vi "PIDRelay.vi"() -> ()   [LabVIEW 2020]
uses:
  <vilib>/Instr/_visa.llb/VISA Configure Serial Port (Instr).vi
  <vilib>/addons/control/pid/NI_PID_pid.lvlib
  <vilib>/addons/control/pid/pid.llb/PID (DBL).vi
panel:
  in  "setpoint":dbl format="%.2f"
  in  "process variable":dbl format="%.2f"
  in  "PID gains":T1={"proportional gain (Kc)"=1.0, "integral time (Ti, min)"=0.01, "derivative time (Td, min)"=0.0} {"derivative time (Td, min)" format="%.3f"; "integral time (Ti, min)" format="%.3f"; "proportional gain (Kc)" format="%.3f"}
  in  "dt (s)":dbl=-1.0 format="%.3f"
  in  "output range":cluster{"output high":dbl, "output low":dbl}={"output high"=100.0, "output low"=-100.0} {"output low" format="%.2f"; "output high" format="%.2f"}
  in  "VISA resource name 2":refnum<visa-resource-name>
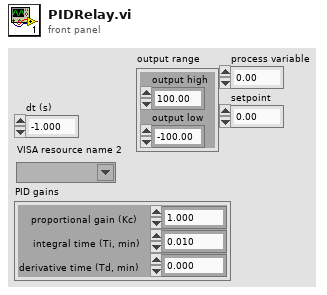
[diagram p1: front panel]
types:
  T1 = cluster{"proportional gain (Kc)":dbl, "integral time (Ti, min)":dbl, "derivative time (Td, min)":dbl}
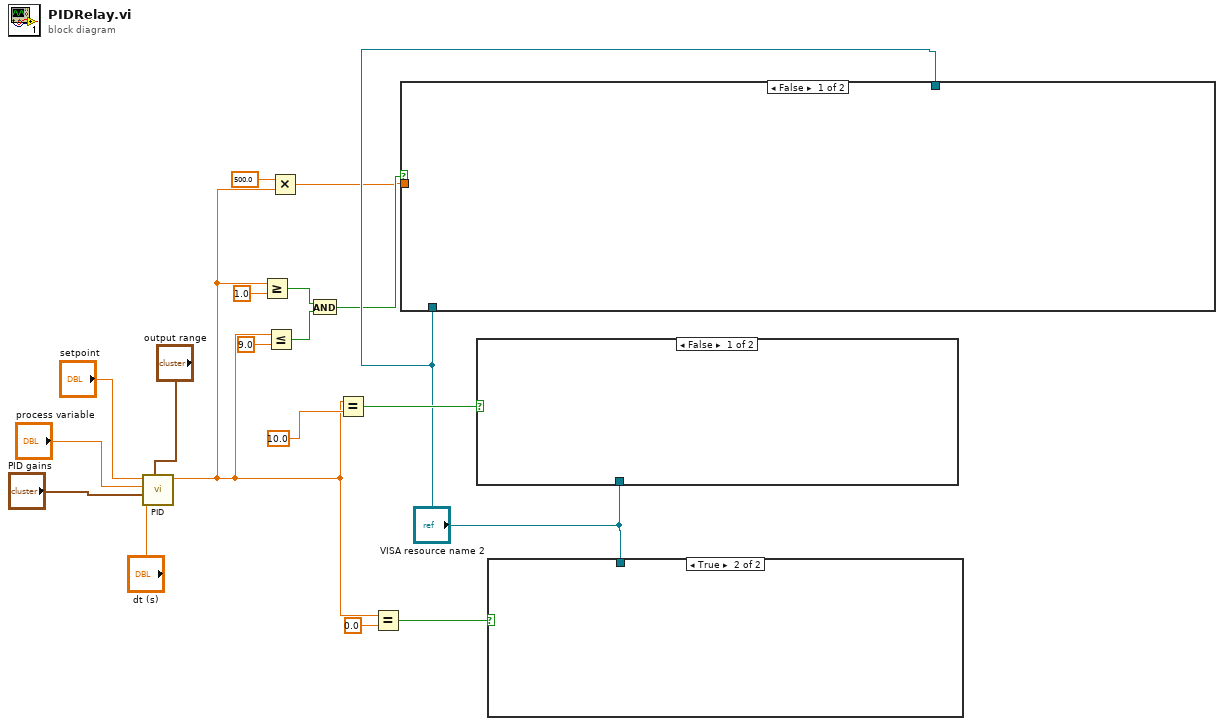
[diagram p0: block diagram]
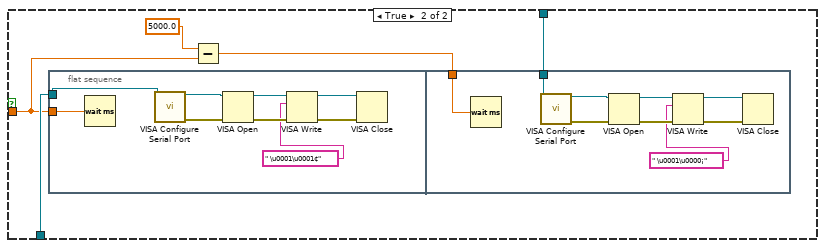
[diagram p2: hidden frame]
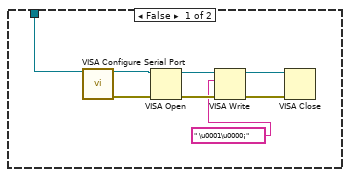
[diagram p3: hidden frame]
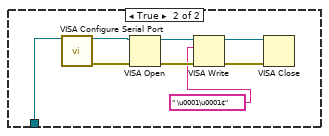
[diagram p4: hidden frame]
diagram:
  n1 = call-poly <vilib>:"PID.vi"("output range"="output range", "dt (s)"="dt (s)", "PID gains"="PID gains", "process variable"="process variable", "setpoint"="setpoint") -> ("output"=w3:dbl)  [unwired: 5 in, 1 out]
  n2 = Greater Or Equal?(x=w3, y=1.0) -> (x >= y?=w8:bool)
  n3 = Less Or Equal?(x=w3, y=9.0) -> (x <= y?=w7:bool)
  n4 = Multiply(x=500.0, y=w3) -> (x*y=w2:dbl)
  n5 = And(x=w8, y=w7) -> (x .and. y?=w6:bool)
  n6 = Equal?(x=w3, y=10.0) -> (x = y?=w18:bool)
  n7 = Equal?(x=w3, y=0.0) -> (x = y?=w17:bool)
  n8 = case shown="False" w6 {
    tunnel: "VISA resource name 2" -> [_ w23]
    tunnel: "VISA resource name 2" -> [_ w22]
    tunnel: w2 -> [_ w19]
    frame False {
    }
    frame True {
      n9 = flat-sequence {
        tunnel: w23 -> [w25]
        tunnel: w19 -> [w24]
        tunnel: w22 -> [w34]
        tunnel: w21 -> [w33]
        frame #0 {
          n10 = Wait (ms)(milliseconds to wait=w24) -> ()  [unwired: 1 out]
          n11 = call-poly "VISA Configure Serial Port"("VISA resource name"=w25) -> ("VISA resource name out"=w32:refnum<visa-resource-name>, "error out"=w31:errorcluster)  [unwired: 13 in]
          n12 = VISA Open(error in (no error)=w31, VISA resource name=w32) -> (VISA resource name=w30:refnum<visa-resource-name>, error out=w29:errorcluster)  [unwired: 3 in]
          n13 = VISA Write(VISA resource name=w30, write buffer=" \u0001\u0001¢", error in (no error)=w29) -> (VISA resource name out=w28:refnum<visa-resource-name>, error out=w27:errorcluster)  [unwired: 1 out]
          n14 = VISA Close(VISA resource name=w28, error in (no error)=w27) -> ()  [unwired: 1 out]
        }
        frame #1 {
          n15 = Wait (ms)(milliseconds to wait=w33) -> ()  [unwired: 1 out]
          n16 = call-poly "VISA Configure Serial Port"("VISA resource name"=w34) -> ("VISA resource name out"=w36:refnum<visa-resource-name>, "error out"=w37:errorcluster)  [unwired: 13 in]
          n17 = VISA Open(error in (no error)=w37, VISA resource name=w36) -> (VISA resource name=w38:refnum<visa-resource-name>, error out=w39:errorcluster)  [unwired: 3 in]
          n18 = VISA Write(VISA resource name=w38, write buffer=" \u0001\u0000¡", error in (no error)=w39) -> (VISA resource name out=w40:refnum<visa-resource-name>, error out=w41:errorcluster)  [unwired: 1 out]
          n19 = VISA Close(VISA resource name=w40, error in (no error)=w41) -> ()  [unwired: 1 out]
        }
      }
      n20 = Subtract(x=5000.0, y=w19) -> (x-y=w21:dbl)
    }
  }
  n21 = case shown="False" w18 {
    tunnel: "VISA resource name 2" -> [_ w42]
    frame False {
    }
    frame True {
      n22 = call-poly "VISA Configure Serial Port"("VISA resource name"=w42) -> ("VISA resource name out"=w49:refnum<visa-resource-name>, "error out"=w48:errorcluster)  [unwired: 13 in]
      n23 = VISA Open(error in (no error)=w48, VISA resource name=w49) -> (VISA resource name=w47:refnum<visa-resource-name>, error out=w46:errorcluster)  [unwired: 3 in]
      n24 = VISA Write(VISA resource name=w47, write buffer=" \u0001\u0001¢", error in (no error)=w46) -> (VISA resource name out=w45:refnum<visa-resource-name>, error out=w44:errorcluster)  [unwired: 1 out]
      n25 = VISA Close(VISA resource name=w45, error in (no error)=w44) -> ()  [unwired: 1 out]
    }
  }
  n26 = case shown="True" w17 {
    tunnel: "VISA resource name 2" -> [w50 _]
    frame False {
      n27 = call-poly "VISA Configure Serial Port"("VISA resource name"=w50) -> ("VISA resource name out"=w57:refnum<visa-resource-name>, "error out"=w56:errorcluster)  [unwired: 13 in]
      n28 = VISA Open(error in (no error)=w56, VISA resource name=w57) -> (VISA resource name=w55:refnum<visa-resource-name>, error out=w54:errorcluster)  [unwired: 3 in]
      n29 = VISA Write(VISA resource name=w55, write buffer=" \u0001\u0000¡", error in (no error)=w54) -> (VISA resource name out=w53:refnum<visa-resource-name>, error out=w52:errorcluster)  [unwired: 1 out]
      n30 = VISA Close(VISA resource name=w53, error in (no error)=w52) -> ()  [unwired: 1 out]
    }
    frame True {
    }
  }
